vi "rqcBob Main Operation SM (FPGA).vi"(0 "Main Operation Parameters":T4, 1 "clock in":bool, 2 "reset":bool, 5 "initiate":bool, 9 "trigger":bool) -> (4 "HW state":T1, 6 "rqcBob Main State":T2={"state"=enum."ready for trigger", "trains generated"=0, "current period"=0, "pulses generated"=0}, 13 "done":bool, 14 "detector.reset":bool)   [LabVIEW 2018]
uses:
  Custom Controls/Main State Machine/rqcBob Main Operation Parameters.ctl
  Custom Controls/Pulse Train/rqcBob Pulse Train Config.ctl
  Custom Controls/Pulse Train/rqcBob Pulse Train.Generation Mode.ctl
  Custom Controls/Pulse Train/rqcBob Pulse Train.First Pulse Delay Mode.ctl
  Custom Controls/rqcBob Modulator Config.ctl
  Custom Controls/rqcBob Window Config.ctl
  Custom Controls/Main State Machine/rqcBob Main SM.ctl
  Custom Controls/Main State Machine/rqcBob Main Operation State.ctl
  Custom Controls/rqcBob HW Control.ctl
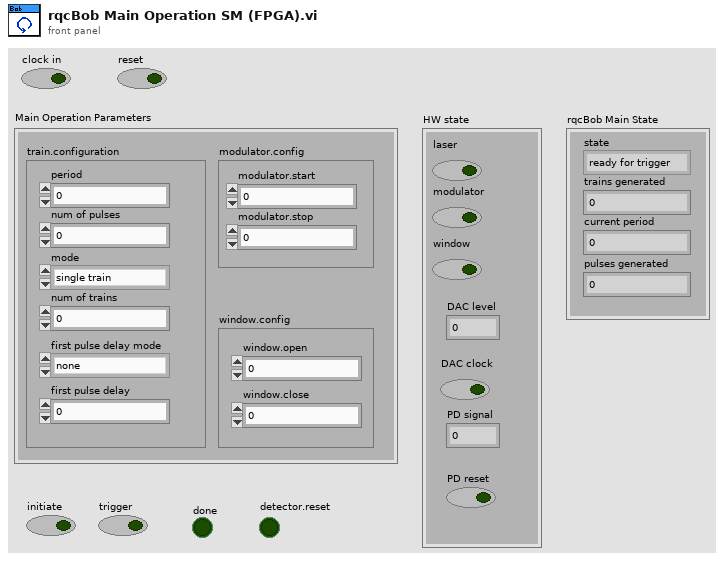
[diagram p1: front panel]
types:
  T1 = typedef "rqcBob HW Control.ctl" = cluster{"laser":bool, "modulator":bool, "window":bool, "DAC level":u8, "DAC clock":bool, "PD signal":u8, "PD reset":bool}
  T2 = typedef "rqcBob Main SM.ctl" = cluster{"state":T3, "trains generated":u16, "current period":u16, "pulses generated":u16}
  T3 = typedef "rqcBob Main Operation State.ctl" = enum8{"idle", "reset", "ready for trigger", "first puls delay", "generate", "end of train"}
  T4 = typedef "rqcBob Main Operation Parameters.ctl" = cluster{"train.configuration":T5, "modulator.config":T8, "window.config":T9}
  T5 = typedef "rqcBob Pulse Train Config.ctl" = cluster{"period":u16, "num of pulses":u16, "mode":T6, "num of trains":u16, "first pulse delay mode":T7, "first pulse delay":u16}
  T6 = typedef "rqcBob Pulse Train.Generation Mode.ctl" = enum8{"single train", "train sequence.single", "train sequence.wait for trigger", "continuous"}
  T7 = typedef "rqcBob Pulse Train.First Pulse Delay Mode.ctl" = enum8{"none", "every train", "first train"}
  T8 = typedef "rqcBob Modulator Config.ctl" = cluster{"modulator.start":u16, "modulator.stop":u16}
  T9 = typedef "rqcBob Window Config.ctl" = cluster{"window.open":u16, "window.close":u16}
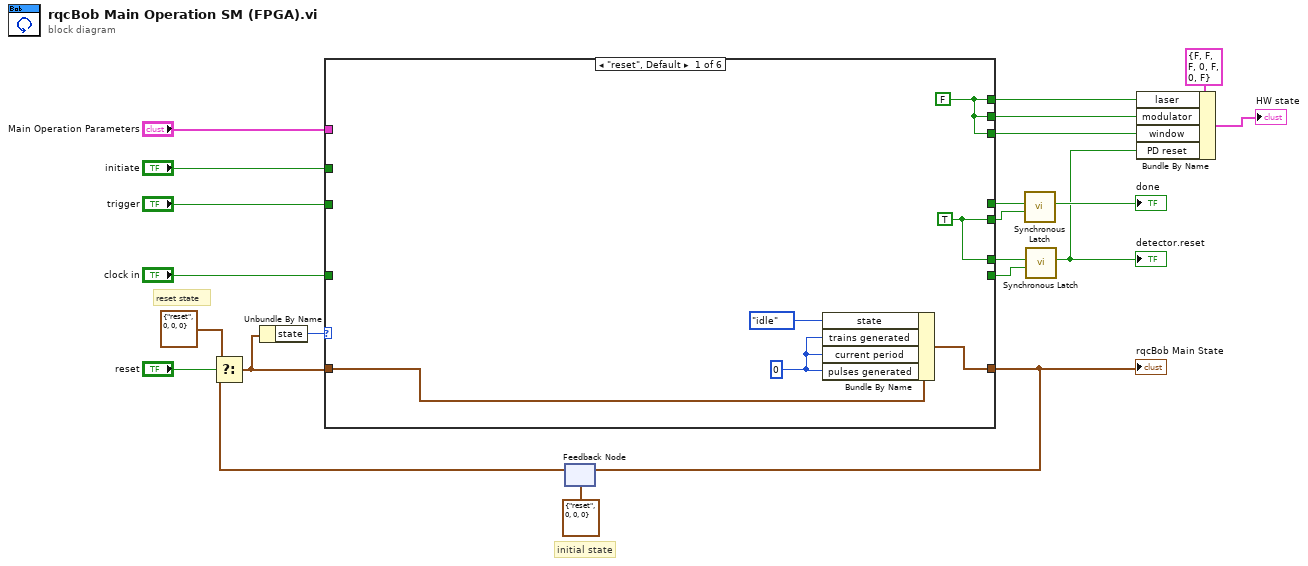
[diagram p0: block diagram]
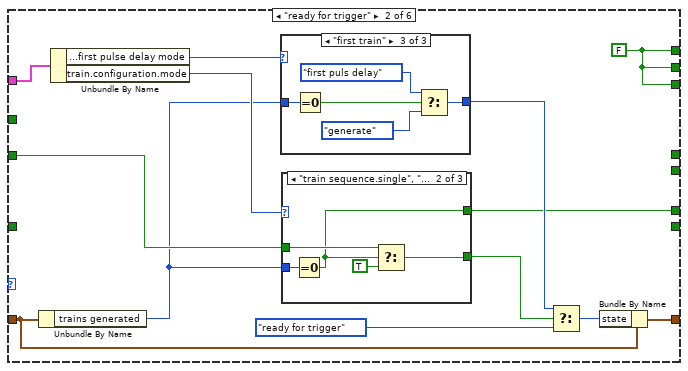
[diagram p2: hidden frame]
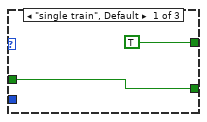
[diagram p3: hidden frame]
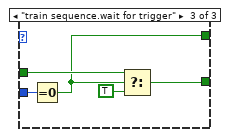
[diagram p4: hidden frame]
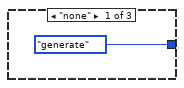
[diagram p5: hidden frame]
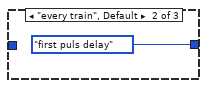
[diagram p6: hidden frame]
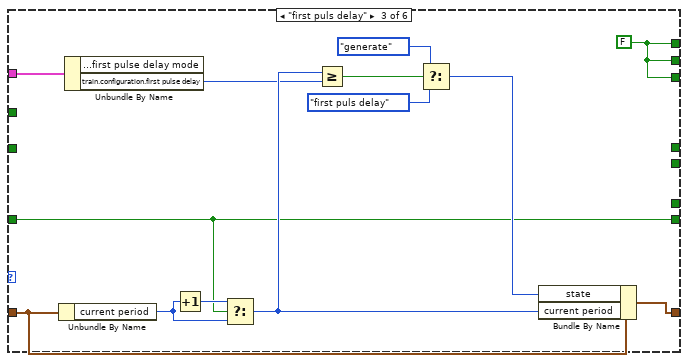
[diagram p7: hidden frame]
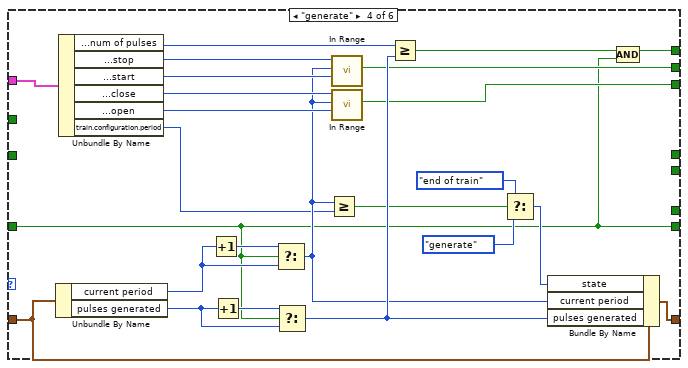
[diagram p8: hidden frame]
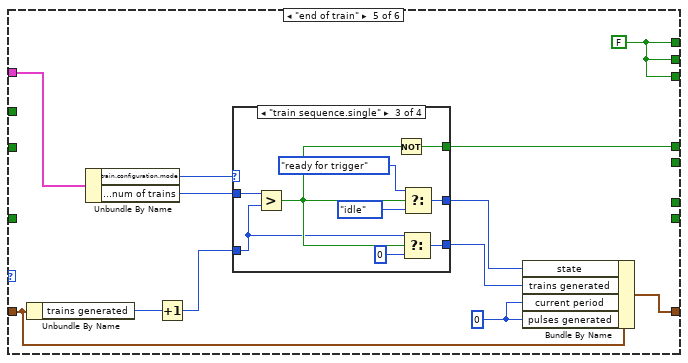
[diagram p9: hidden frame]
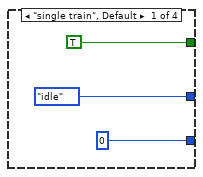
[diagram p10: hidden frame]
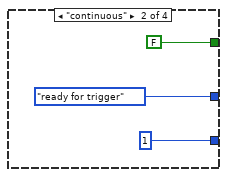
[diagram p11: hidden frame]
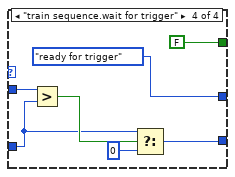
[diagram p12: hidden frame]
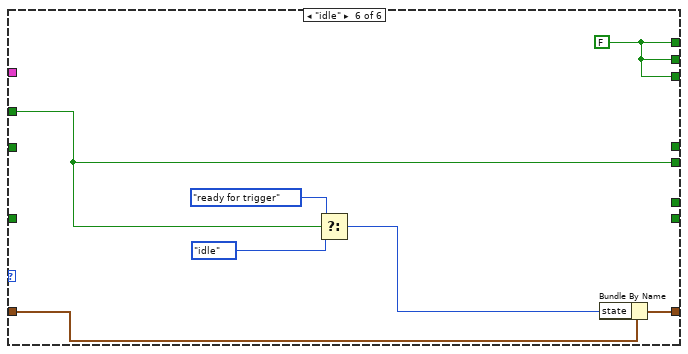
[diagram p13: hidden frame]
diagram:
  # "reset state"
  # "initial state"
  n1 = feedback #1(T2 {"state"=enum."reset", "trains generated"=0, "current period"=0, "pulses generated"=0} ("rqcBob Main SM")) -> (w19:T2)
  n2 = Select(t=T2 {"state"=enum."reset", "trains generated"=0, "current period"=0, "pulses generated"=0} ("rqcBob Main SM"), s="reset", f=w19) -> (s? t:f=w17:T2)
  n3 = Unbundle By Name(w17) -> ("state"=w20:T3)
  n4 = case shown="\"reset\", Default" w20 {
    tunnel: w17 -> [w28 w34 w70 w93 w105 w137]
    tunnel: [w26 w41 w69 w92 w104 w136] -> w18
    tunnel: "clock in" -> [_ _ w61 w74 _ _]
    tunnel: "trigger" -> [_ w32 _ _ _ _]
    tunnel: "Main Operation Parameters" -> [_ w40 w73 w91 w109 _]
    tunnel: [w25 w35 w62 w75 w101 w138] -> w13
    tunnel: [w25 w35 w62 w85 w101 w138] -> w12
    tunnel: [w25 w35 w62 w82 w101 w138] -> w2
    tunnel: "initiate" -> [_ _ _ _ _ w132]
    tunnel: [_ _ _ _ w100 _] -> w9
    tunnel: [w23 _ _ _ _ w132] -> w7
    tunnel: [w23 w31 _ _ _ _] -> w6
    tunnel: [_ _ w61 w74 _ _] -> w5
    frame "reset", Default {
      w23 = TRUE ("laser")
      w24 = u16 0 ("trains generated")
      w25 = FALSE ("laser")
      n5 = Bundle By Name(cluster=w28, "state"=rqcBob_Main_Operation_State."idle", "trains generated"=w24, "current period"=w24, "pulses generated"=w24) -> (w26:T2)
    }
    frame "ready for trigger" {
      w35 = FALSE ("laser")
      n6 = Unbundle By Name(w34) -> ("trains generated"=w30:u16)
      n7 = Unbundle By Name(w40) -> ("train.configuration.first pulse delay mode"=w37:T7, "train.configuration.mode"=w33:T6)
      n8 = case shown="\"first train\"" w37 {
        tunnel: [rqcBob_Main_Operation_State."generate" ("state") rqcBob_Main_Operation_State."first puls delay" ("state") w56] -> w36
        tunnel: w30 -> [_ _ w60]
        frame "none" {
        }
        frame "every train", Default {
        }
        frame "first train" {
          n9 = Equal To 0?(x=w60) -> (x = 0?=w59:bool)
          n10 = Select(t=rqcBob_Main_Operation_State."first puls delay" ("state"), s=w59, f=rqcBob_Main_Operation_State."generate") -> (s? t:f=w56:T3)
        }
      }
      n11 = case shown="\"train sequence.single\", \"continuous\"" w33 {
        tunnel: w32 -> [w43 w47 w52]
        tunnel: [w43 w45 w50] -> w29
        tunnel: [TRUE ("set") w44 w49] -> w31
        tunnel: w30 -> [_ w48 w53]
        frame "single train", Default {
        }
        frame "train sequence.single", "continuous" {
          n12 = Equal To 0?(x=w48) -> (x = 0?=w44:bool)
          n13 = Select(t=w47, s=w44, f=TRUE ("trigger")) -> (s? t:f=w45:bool)
        }
        frame "train sequence.wait for trigger" {
          n14 = Equal To 0?(x=w53) -> (x = 0?=w49:bool)
          n15 = Select(t=w52, s=w49, f=TRUE ("trigger")) -> (s? t:f=w50:bool)
        }
      }
      n16 = Select(t=w36, s=w29, f=rqcBob_Main_Operation_State."ready for trigger" ("state")) -> (s? t:f=w38:T3)
      n17 = Bundle By Name(cluster=w34, "state"=w38) -> (w41:T2)
    }
    frame "first puls delay" {
      w62 = FALSE ("laser")
      n18 = Unbundle By Name(w70) -> ("current period"=w71:u16)
      n19 = Unbundle By Name(w73) -> ("train.configuration.first pulse delay"=w67:u16)  [unwired: 1 out]
      n20 = Increment(x=w71) -> (x+1=w72:u16)
      n21 = Select(t=w72, s=w61, f=w71) -> (s? t:f=w68:u16)
      n22 = Greater Or Equal?(x=w68, y=w67) -> (x >= y?=w66:bool)
      n23 = Select(t=rqcBob_Main_Operation_State."generate" ("state"), s=w66, f=rqcBob_Main_Operation_State."first puls delay") -> (s? t:f=w63:T3)
      n24 = Bundle By Name(cluster=w70, "state"=w63, "current period"=w68) -> (w69:T2)
    }
    frame "generate" {
      n25 = Unbundle By Name(w93) -> ("current period"=w96:u16, "pulses generated"=w94:u16)
      n26 = Unbundle By Name(w91) -> ("train.configuration.num of pulses"=w90:u16, "modulator.config.modulator.stop"=w87:u16, "modulator.config.modulator.start"=w86:u16, "window.config.window.close"=w84:u16, "window.config.window.open"=w83:u16, "train.configuration.period"=w80:u16)
      n27 = Increment(x=w96) -> (x+1=w97:u16)
      n28 = Increment(x=w94) -> (x+1=w95:u16)
      n29 = Select(t=w97, s=w74, f=w96) -> (s? t:f=w81:u16)
      n30 = Select(t=w95, s=w74, f=w94) -> (s? t:f=w89:u16)
      n31 = Greater Or Equal?(x=w81, y=w80) -> (x >= y?=w79:bool)
      n32 = call <vilib>:"In Range.vi"("lower limit"=w86, "x"=w81, "upper limit"=w87) -> ("in range"=w85:bool)  [unwired: 8 in]
      n33 = call <vilib>:"In Range.vi"("lower limit"=w83, "x"=w81, "upper limit"=w84) -> ("in range"=w82:bool)  [unwired: 8 in]
      n34 = Greater Or Equal?(x=w90, y=w89) -> (x >= y?=w88:bool)
      n35 = Select(t=rqcBob_Main_Operation_State."end of train" ("state"), s=w79, f=rqcBob_Main_Operation_State."generate" ("state")) -> (s? t:f=w76:T3)
      n36 = Bundle By Name(cluster=w93, "state"=w76, "current period"=w81, "pulses generated"=w89) -> (w92:T2)
      n37 = Compound Arithmetic op=AND(w88, w74) -> (w75:bool)
    }
    frame "end of train" {
      w101 = FALSE ("laser")
      w103 = u16 0 ("inner period position")
      n38 = Unbundle By Name(w105) -> ("trains generated"=w108:u16)
      n39 = Unbundle By Name(w109) -> ("train.configuration.mode"=w107:T6, "train.configuration.num of trains"=w106:u16)
      n40 = Increment(x=w108) -> (x+1=w99:u16)
      n41 = case shown="\"train sequence.single\"" w107 {
        tunnel: w106 -> [_ _ w124 w131]
        tunnel: [rqcBob_Main_Operation_State."idle" ("f") rqcBob_Main_Operation_State."ready for trigger" ("f") w122 rqcBob_Main_Operation_State."ready for trigger" ("f")] -> w102
        tunnel: [TRUE FALSE w120 FALSE] -> w100
        tunnel: w99 -> [_ _ w116 w127]
        tunnel: [u16 0 ("trains generated") u16 1 ("trains generated") w118 w129] -> w98
        frame "single train", Default {
        }
        frame "continuous" {
        }
        frame "train sequence.single" {
          n42 = Greater?(x=w124, y=w116) -> (0:w119:bool)
          n43 = Not(x=w119) -> (.not. x?=w120:bool)
          n44 = Select(t=w116, s=w119, f=u16 0) -> (s? t:f=w118:u16)
          n45 = Select(t=rqcBob_Main_Operation_State."ready for trigger" ("f"), s=w119, f=rqcBob_Main_Operation_State."idle") -> (s? t:f=w122:T3)
        }
        frame "train sequence.wait for trigger" {
          n46 = Greater?(x=w131, y=w127) -> (0:w130:bool)
          n47 = Select(t=w127, s=w130, f=u16 0) -> (s? t:f=w129:u16)
        }
      }
      n48 = Bundle By Name(cluster=w105, "state"=w102, "trains generated"=w98, "current period"=w103, "pulses generated"=w103) -> (w104:T2)
    }
    frame "idle" {
      w138 = FALSE ("laser")
      n49 = Select(t=rqcBob_Main_Operation_State."ready for trigger" ("state"), s=w132, f=rqcBob_Main_Operation_State."idle" ("state")) -> (s? t:f=w133:T3)
      n50 = Bundle By Name(cluster=w137, "state"=w133) -> (w136:T2)
    }
  }
  "rqcBob Main State" <- w18
  n51 = feedback-in #1(w18) -> ()
  n52 = call <vilib>:"Synchronous Latch.vi"("clear"=w7, "set"=w9) -> ("out"=→"done":bool)  [unwired: 9 in]
  n53 = call <vilib>:"Synchronous Latch.vi"("clear"=w5, "set"=w6) -> ("out"=w1:bool)  [unwired: 9 in]
  "detector.reset" <- w1
  n54 = Bundle By Name(cluster=T1 {"laser"=FALSE, "modulator"=FALSE, "window"=FALSE, "DAC level"=0, "DAC clock"=FALSE, "PD signal"=0, "PD reset"=FALSE} ("rqcBob HW Control"), "laser"=w13, "modulator"=w12, "window"=w2, "PD reset"=w1) -> (→"HW state":T1)
